vi "SSH Smart Open Session.vi"(7 "Force Reconnect?":bool, 8 "Error In":errorcluster, 11 "Install LV Data in":T1={"SSH Session"=refnum, "Status Log"="", "Detailed Log"="", "Credentials"={"Hostname or IP"="192.168.7.2", "Username"="root", "Password"=""}, "Target Info"={"OS Version"="", "CPU"="", "Systemd Version"="", "Internet Access"=FALSE, "Device Type"="", "LV Installed Ver"="", "LV Available Ver"="", "LV Upgrade Available"=FALSE, "Hostname"="", "NIC Info"=[]}, "Reboot Required?"=FALSE}) -> (0 "Error Out":errorcluster, 1 "Status":string, 2 "Connected?":bool, 3 "Install LV Data out":T1={"SSH Session"=refnum, "Status Log"="", "Detailed Log"="", "Credentials"={"Hostname or IP"="192.168.7.2", "Username"="root", "Password"=""}, "Target Info"={"OS Version"="", "CPU"="", "Systemd Version"="", "Internet Access"=FALSE, "Device Type"="", "LV Installed Ver"="", "LV Available Ver"="", "LV Upgrade Available"=FALSE, "Hostname"="", "NIC Info"=[]}, "Reboot Required?"=FALSE})   [LabVIEW 2014, in "LMH-LINX.lvlib"]
uses:
  <vilib>/MakerHub/LINX/LMH-LINX.lvlib
  <vilib>/MakerHub/LINX/Private/Utilties/Target Management/Install LV Data.ctl
  C:/Program Files (x86)/National Instruments/LabVIEW 2014/vi.lib/MakerHub/LINX/Resources/Renci.SshNet.dll
  Resources/Renci.SshNet.dll
  <vilib>/MakerHub/LINX/Private/Utilties/Target Management/Target Info.ctl
  <vilib>/MakerHub/LINX/Private/Utilties/Target Management/NIC Info.ctl
  <vilib>/MakerHub/LINX/Private/Utilties/Target Management/NIC Mode.ctl
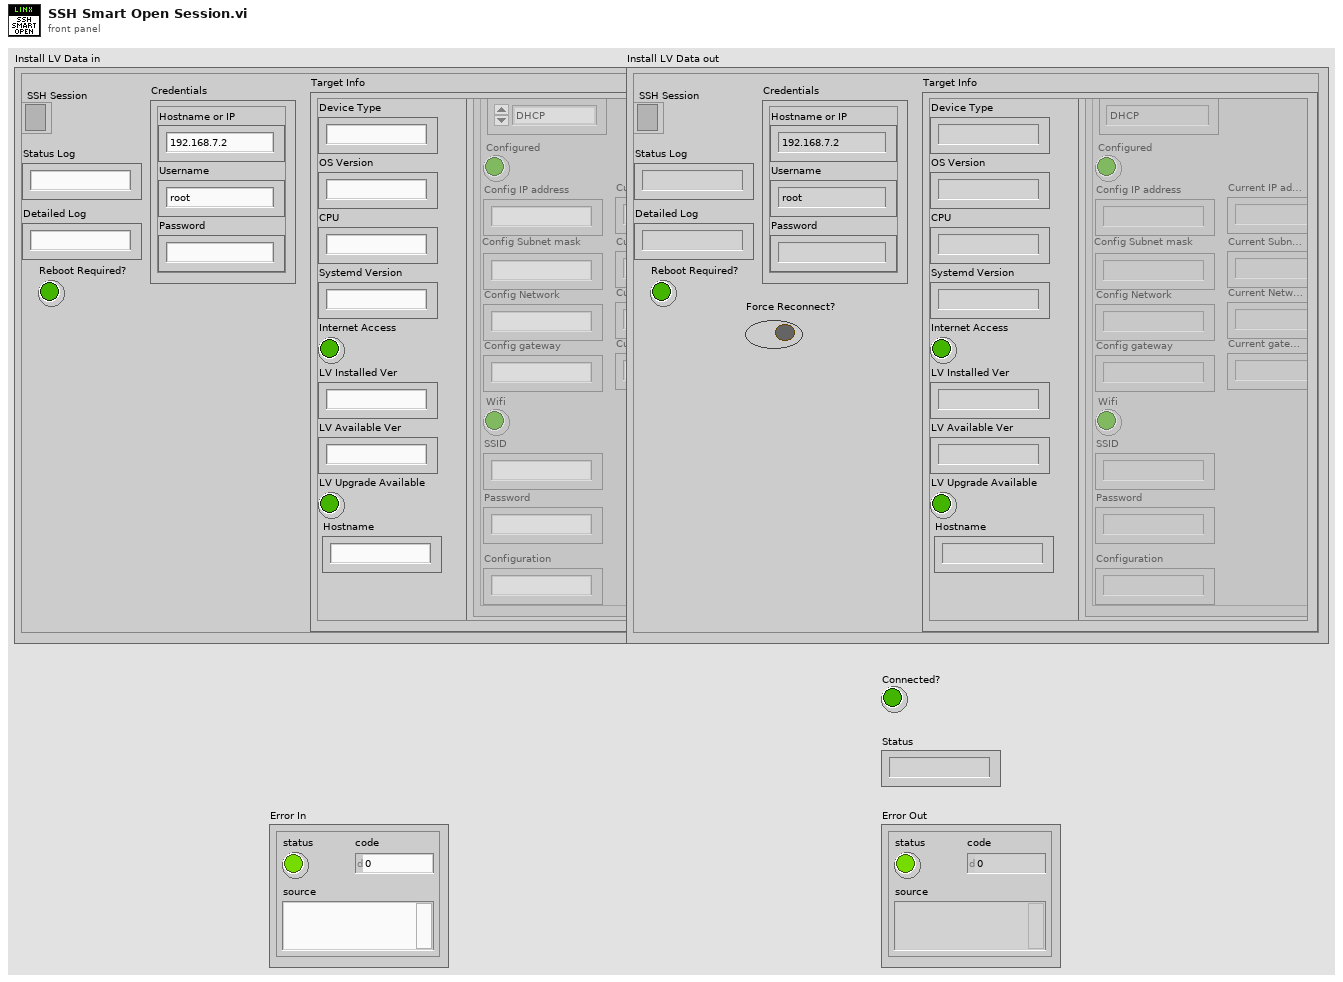
[diagram p1: front panel]
types:
  T1 = typedef "LMH-LINX.lvlib/Install LV Data.ctl" = cluster{"SSH Session":refnum<k24>, "Status Log":string, "Detailed Log":string, "Credentials":cluster{"Hostname or IP":string, "Username":string, "Password":string}, "Target Info":T2, "Reboot Required?":bool}
  T2 = typedef "LMH-LINX.lvlib/Target Info.ctl" = cluster{"OS Version":string, "CPU":string, "Systemd Version":string, "Internet Access":bool, "Device Type":string, "LV Installed Ver":string, "LV Available Ver":string, "LV Upgrade Available":bool, "Hostname":string, "NIC Info":T3[]}
  T3 = typedef "LMH-LINX.lvlib/NIC Info.ctl" = cluster{"Name":string, "NIC Mode":T4, "Configured":bool, "Config IP address":string, "Config Subnet mask":string, "Config Network":string, "Config gateway":string, "Wifi":bool, "SSID":string, "Password":string, "Configuration":string, "Current IP address":string, "Current Subnet mask":string, "Current gateway":string, "Current Network":string}
  T4 = typedef "LMH-LINX.lvlib/NIC Mode.ctl" = enum16{"DHCP", "Static", "Loopback"}
  T5 = cluster{"Hostname or IP":string, "Username":string, "Password":string}
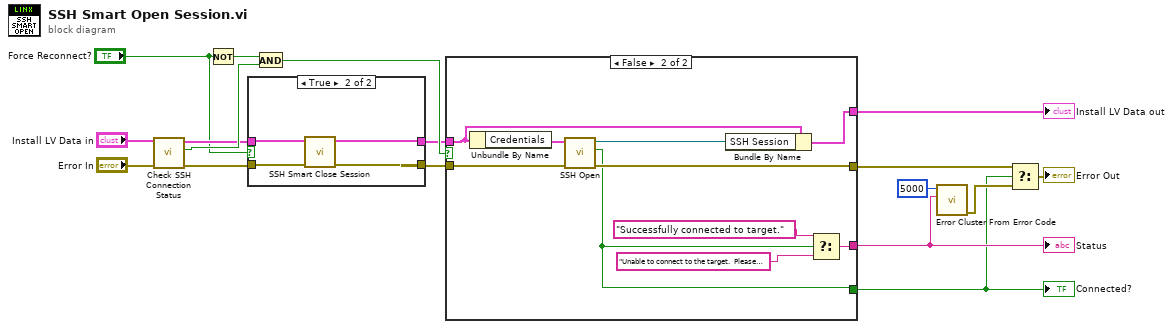
[diagram p0: block diagram]
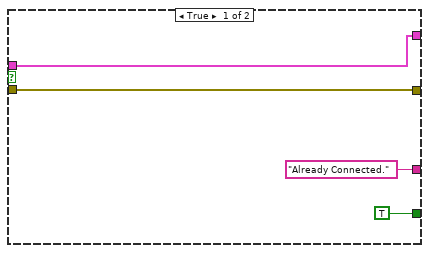
[diagram p3: hidden frame]
diagram:
  n1 = call <vilib>:"Check SSH Connection Status.vi"("Error In"="Error In", "Install LV Data in"="Install LV Data in") -> ("Error Out"=w5:errorcluster, "IsConnected"=w6:bool, "Install LV Data"=w3:T1)  [unwired: 7 in]
  n2 = Not(x="Force Reconnect?") -> (.not. x?=w8:bool)
  n3 = case shown="True" "Force Reconnect?" {
    tunnel: w5 -> [w19 w23]
    tunnel: [w19 w22] -> w4
    tunnel: w3 -> [w18 w20]
    tunnel: [w18 w21] -> w2
    frame False {
    }
    frame True {
      n4 = call <vilib>:"SSH Smart Close Session.vi"("Error In"=w23, "Install LV Data"=w20) -> ("Error Out"=w22:errorcluster, "Install LV Data"=w21:T1)  [unwired: 8 in]
    }
  }
  n5 = And(x=w8, y=w6) -> (x .and. y?=w7:bool)
  n6 = case shown="False" w7 {
    tunnel: [w25 w37] -> w10
    tunnel: ["Already Connected." w35] -> w13
    tunnel: [TRUE ("Connected?") w34] -> w11
    tunnel: w4 -> [w25 w33]
    tunnel: [w24 w32] -> w15
    tunnel: w2 -> [w24 w30]
    frame True {
    }
    frame False {
      n7 = Unbundle By Name(w30) -> ("Credentials"=w29:T5)
      n8 = call <vilib>:"SSH Open.vi"("Error In"=w33, "Credentials"=w29) -> ("Error Out"=w37:errorcluster, "Connected?"=w34:bool, "SSH Session"=w31:refnum<k24>)  [unwired: 7 in]
      n9 = Bundle By Name(cluster=w30, "SSH Session"=w31) -> (w32:T1)
      n10 = Select(t="Successfully connected to target.", s=w34, f="Unable to connect to the target.  Please make sure the specified Hostname/IP, Username and Password are correct and try again.  If this problem persists please search then create a thread on the Makerhub forums at labviewmakerhub.com/forums/linx.") -> (s? t:f=w35:string)
    }
  }
  "Status" <- w13
  "Install LV Data out" <- w15
  "Connected?" <- w11
  n11 = call <vilib>:"Error Cluster From Error Code.vi"("error message (\"\")"=w13, "error code (0)"=5000) -> ("error out"=w12:errorcluster)  [unwired: 7 in]
  n12 = Select(t=w10, s=w11, f=w12) -> (s? t:f=→"Error Out":errorcluster)
